vi "Get RemIO UI Ref.vi"(8 "error in (no error)":errorcluster, 11 "11102 in":refnum<class "11102.lvclass">) -> (0 "error out":errorcluster, 2 "VI Refnum":refnum<vi>, 3 "11102 out":refnum<class "11102.lvclass">)   [LabVIEW 2020, in "Modules.lvlib" / "11102.lvclass"]
uses:
  11102.lvclass
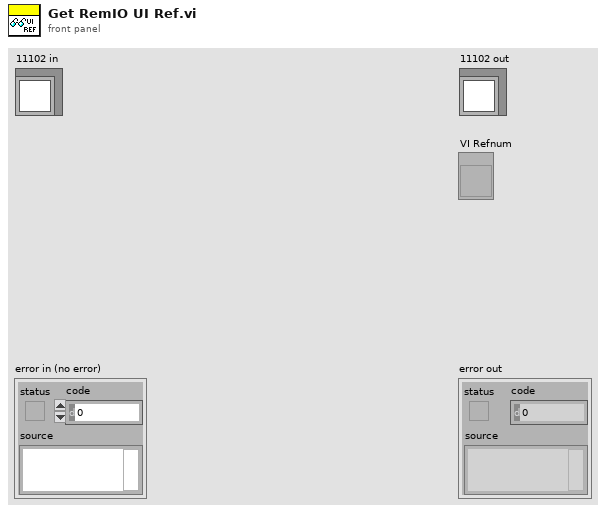
[diagram p1: front panel]
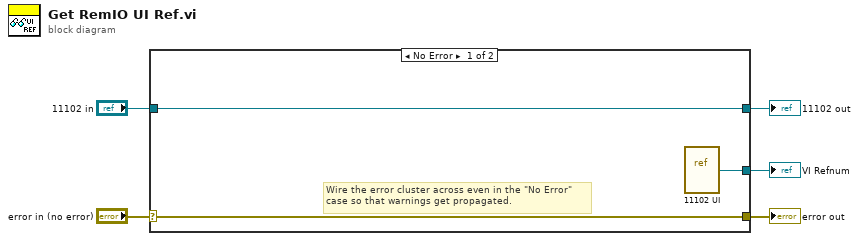
[diagram p0: block diagram]
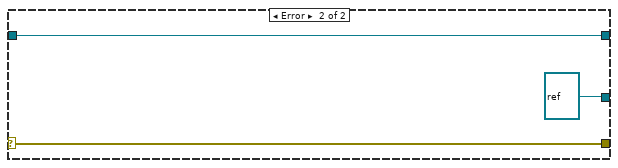
[diagram p2: hidden frame]
diagram:
  n1 = case shown="No Error" "error in (no error)" {
    selector: "error in (no error)" -> [w7 w11]
    tunnel: [w7 w11] -> w2
    tunnel: [w8 w10] -> w4
    tunnel: "11102 in" -> [w8 w10]
    tunnel: [w6 refnum<vi> refnum] -> w5
    frame No Error {
      # "Wire the error cluster across even in the \"No Error\"\ncase so that warnings get propagated."
      n2 = vi-ref "11102 UI.vi"() -> (w6:refnum<vi>)
    }
    frame Error {
    }
  }
  "error out" <- w2
  "11102 out" <- w4
  "VI Refnum" <- w5
